vi "PH_BL-Master.set vacuum Gui element tip strips.vi"(0 "i ref in":refnum<vi>, 5 "error in (no error)":errorcluster) -> (14 "i ref out":refnum<vi>, 19 "error out":errorcluster)   [LabVIEW 2014, in "PH_BL-Master.lvlib"]
doc: "Within this VI the tip strips of the VACUUM GUI elements are set."
uses:
  PH_BL-Master.lvlib
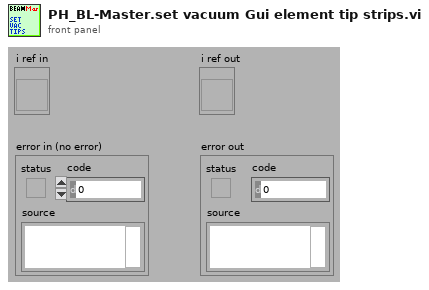
[diagram p1: front panel]
types:
  T1 = typedef "PH_BL-Master.lvlib/PH_BL-Master.i attribute.ctl" = cluster{"Remote controlled":bool, "Boolean Condition Service Subscriber":refnum<vi>[], "Picture Condition Service Subscriber":refnum<vi>[], "R2S":cluster{"GUI Ref":refnum<vi>, "State":bool}, "Vacua":cluster{"GUI Ref":refnum<vi>, "Limit":dbl, "Curr Value":dbl, "in range":bool}[], "O2 Inspection":cluster{"GUI Ref":refnum<vi>, "Concentration":dbl, "State":T2}[], "Boolean Status Service Subscriber":cluster{"GUI Ref":refnum<vi>, "Status":T2, "no Link?":bool, "Status Subscriber Class":T3}[], "Picture Status Service Subscriber":cluster{"GUI Ref":refnum<vi>, "Status":T2, "no Link?":bool, "Status Subscriber Class":T3}[], "6P 4Q Service Subscriber":cluster{"GUI Ref":refnum<vi>, "Selector":T4, "no Link?":bool}[], "Index of latest 6P 4Q changing Instance":i32, "Index of latest Picture Status changing Instance":i32, "Index of latest Boolean Status changing Instance":i32, "Vision ID on same Node":string, "Start Phase over?":bool, "GUI Ref Delete":refnum<vi>}
  T2 = typedef "PH_StatusHandler.lvlib/PH_StatusHandler.Status.ctl" = i16
  T3 = typedef "PH_BL-Master.lvlib/PH_BL-Master.Status Subscriber Class.ctl" = enum16{"unknown", "Switch", "BB", "6P Switch", "Switch GUI", "Switch and 6P State", "Force Sensor"}
  T4 = typedef "PH_4_Pos_Selector.lvlib/PH_4_Pos_Selector.Position Selector.ctl" = u16
  T5 = cluster{"GUI Ref":refnum<vi>, "Limit":dbl, "Curr Value":dbl, "in range":bool}[]
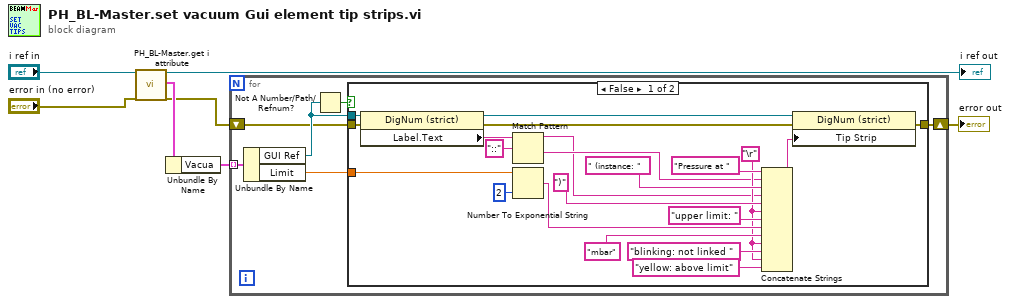
[diagram p0: block diagram]
diagram:
  n1 = call "PH_BL-Master.get i attribute.vi"("i ref in"="i ref in", "error in (no error)"="error in (no error)") -> ("i ref out"=→"i ref out":refnum<vi>, "i attribute"=w7:T1, "error out"=w2:errorcluster)  [unwired: 15 in]
  n2 = Unbundle By Name(w7) -> ("Vacua"=w3:T5)
  n3 = for {
    shift-right: [w11] -> w1
    shift-left: w2 -> [w9]
    tunnel: w3 -> [w10] mode=indexing
    n4 = Unbundle By Name(w10) -> ("GUI Ref"=w13:refnum<vi>, "Limit"=w12:dbl)
    n5 = Not A Number/Path/Refnum?(number/path/refnum=w13) -> (NaN/Path/Refnum?=w8:bool)
    n6 = case shown="False" w8 {
      tunnel: w13 -> [w26 _]
      tunnel: w12 -> [w23 _]
      tunnel: [w21 w35] -> w11
      tunnel: w9 -> [w19 w35]
      frame False {
        w24 = "\r"
        n7 = property class="DigNum (strict)"(reference=w26, error in=w19) -> (reference out=w20:refnum<vi>, error out=w18:errorcluster, "Label.Text"=w17:string)
        n8 = Match Pattern(string=w17, regular expression="::") -> (before substring=w14:string, after substring=w15:string)  [unwired: 1 in, 2 out]
        n9 = Number To Exponential String(number=w23, precision (6)=i16 2) -> (E-format string=w34:string)  [unwired: 2 in]
        n10 = Concatenate Strings("Pressure at " ("string"), w15, " (instance: " ("string"), w14, ")" ("string"), w24, "upper limit: " ("string"), w34, "mbar" ("string"), w24, "blinking: not linked " ("string"), w24, "yellow: above limit" ("string")) -> (w25:string)
        n11 = property class="DigNum (strict)"(reference=w20, error in=w18, "Tip Strip"=w25) -> (error out=w21:errorcluster)  [unwired: 1 out]
      }
      frame True {
      }
    }
  }
  "error out" <- w1
